vi "Convert MBR to Degrees Minutes Seconds.vi"(11 ".shp header":T1 {"MBR min Y" format="%#.7g"; "MBR max Y" format="%#.7g"; "MBR max X" format="%#.7g"; "MBR min X" format="%#.7g"}) -> (3 "MBR in DMS":T2 {"MaxY Sec" format="%#.5g"; "MaxY Min" format="%#.5g"; "MaxY Deg" format="%#.5g"; "MaxX Sec" format="%#.5g"; "MaxX Min" format="%#.5g"; "MaxX Deg" format="%#.5g"; "MinY Sec" format="%#.5g"; "MinY Min" format="%#.5g"; "MinY Deg" format="%#.5g"; "MinX Sec" format="%#.5g"; "MinX Min" format="%#.5g"; "MinX Deg" format="%#.5g"})   [LabVIEW 2014]
uses:
  Control/MBR DMS.ctl
  Control/SHP SHX Header.ctl
  Sub VI/Decimal to Degrees Minutes Seconds.vi
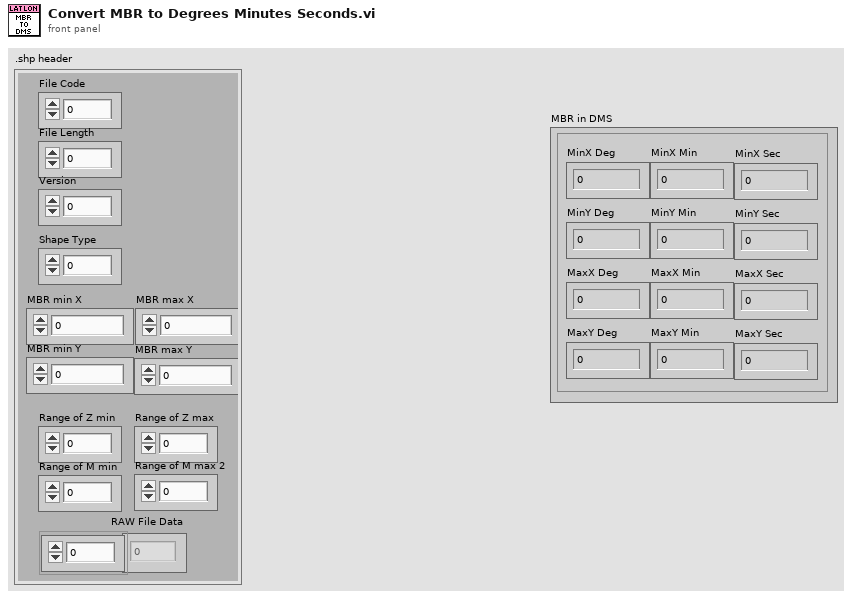
[diagram p1: front panel]
types:
  T1 = typedef "SHP SHX Header.ctl" = cluster{"File Code":i32, "File Length":i32, "Version":i32, "Shape Type":i32, "MBR min X":dbl, "MBR max X":dbl, "MBR max Y":dbl, "Range of Z min":dbl, "Range of Z max":dbl, "Range of M min":dbl, "Range of M max 2":dbl, "MBR min Y":dbl, "RAW File Data":u8[]}
  T2 = typedef "MBR DMS.ctl" = cluster{"MinX Deg":dbl, "MinX Min":dbl, "MinX Sec":dbl, "MinY Deg":dbl, "MinY Min":dbl, "MinY Sec":dbl, "MaxX Deg":dbl, "MaxX Min":dbl, "MaxX Sec":dbl, "MaxY Deg":dbl, "MaxY Min":dbl, "MaxY Sec":dbl}
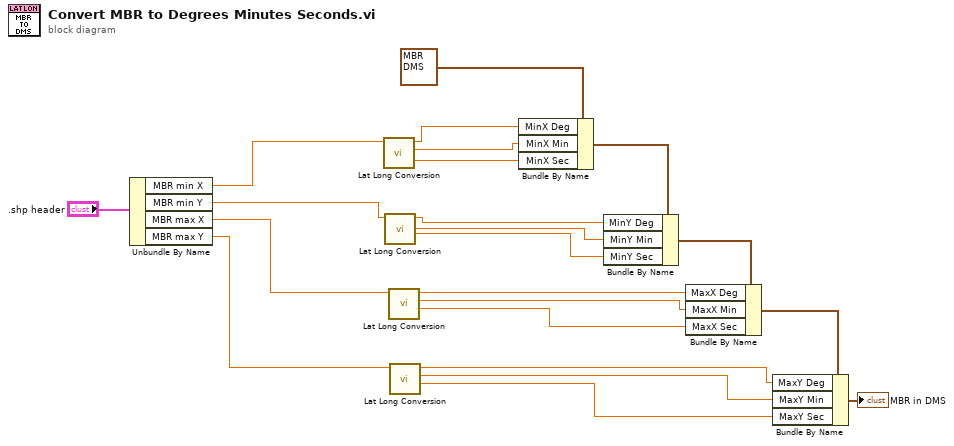
[diagram p0: block diagram]
diagram:
  n1 = Unbundle By Name(".shp header") -> ("MBR min X"=w21:dbl, "MBR min Y"=w20:dbl, "MBR max X"=w19:dbl, "MBR max Y"=w18:dbl)
  n2 = call-poly "Lat Long Conversion.vi"("Lat Long Input (decimal)"=w21) -> ("Seonds"=w14:dbl, "Minutes"=w15:dbl, "Degrees"=w16:dbl)  [unwired: 8 in]
  n3 = call-poly "Lat Long Conversion.vi"("Lat Long Input (decimal)"=w20) -> ("Seonds"=w10:dbl, "Minutes"=w11:dbl, "Degrees"=w12:dbl)  [unwired: 8 in]
  n4 = call-poly "Lat Long Conversion.vi"("Lat Long Input (decimal)"=w19) -> ("Seonds"=w6:dbl, "Minutes"=w7:dbl, "Degrees"=w8:dbl)  [unwired: 8 in]
  n5 = call-poly "Lat Long Conversion.vi"("Lat Long Input (decimal)"=w18) -> ("Seonds"=w2:dbl, "Minutes"=w3:dbl, "Degrees"=w4:dbl)  [unwired: 8 in]
  n6 = Bundle By Name(cluster=T2 {"MinX Deg"=0.0, "MinX Min"=0.0, "MinX Sec"=0.0, "MinY Deg"=0.0, "MinY Min"=0.0, "MinY Sec"=0.0, "MaxX Deg"=0.0, "MaxX Min"=0.0, "MaxX Sec"=0.0, "MaxY Deg"=0.0, "MaxY Min"=0.0, "MaxY Sec"=0.0} ("MBR in DMS"), "MinX Deg"=w16, "MinX Min"=w15, "MinX Sec"=w14) -> (w13:T2)
  n7 = Bundle By Name(cluster=w13, "MinY Deg"=w12, "MinY Min"=w11, "MinY Sec"=w10) -> (w9:T2)
  n8 = Bundle By Name(cluster=w9, "MaxX Deg"=w8, "MaxX Min"=w7, "MaxX Sec"=w6) -> (w5:T2)
  n9 = Bundle By Name(cluster=w5, "MaxY Deg"=w4, "MaxY Min"=w3, "MaxY Sec"=w2) -> (→"MBR in DMS":T2)
